vi "Set Double Complex.vi"(8 "error in":errorcluster, 9 "value":cdb, 10 "variable name":string, 11 "GOLPI ref. in":T1={"pipe handle"={"lv_proc.dll file path"=path "", "process instance handle"=[], "debug mode"=FALSE, "debug data"=[]}, "fast read timeout [ms]"=500, "fast read settle time [ms]"=10, "fast read to multiple [ms]"=1, "max elements per input line"=100, "slow read timeout [ms]"=5000, "stdin double format specifier"="%_16e", "max elements per stdout output column"=100, "console mode bitstream"=FALSE, "bitstream first read timeout [ms]"=1000, "bitstream read timeout [ms]"=50, "struct transfer possible"=FALSE, "matlab mode"=FALSE, "var pipe write timeout [ms]"=5000, "variable pipe mode"=FALSE, "variable pipe buffer size [Bytes]"=10000000, "variable pipe block size [Bytes]"=1000000} {"variable pipe block size [Bytes]" format="%.0p"; "variable pipe buffer size [Bytes]" format="%.0p"}) -> (0 "error out":errorcluster, 3 "GOLPI ref. out":T1={"pipe handle"={"lv_proc.dll file path"=path "", "process instance handle"=[], "debug mode"=FALSE, "debug data"=[]}, "fast read timeout [ms]"=500, "fast read settle time [ms]"=10, "fast read to multiple [ms]"=1, "max elements per input line"=100, "slow read timeout [ms]"=5000, "stdin double format specifier"="%_16e", "max elements per stdout output column"=100, "console mode bitstream"=FALSE, "bitstream first read timeout [ms]"=1000, "bitstream read timeout [ms]"=50, "struct transfer possible"=FALSE, "matlab mode"=FALSE, "var pipe write timeout [ms]"=5000, "variable pipe mode"=FALSE, "variable pipe buffer size [Bytes]"=10000000, "variable pipe block size [Bytes]"=1000000} {"variable pipe block size [Bytes]" format="%.0p"; "variable pipe buffer size [Bytes]" format="%.0p"})   [LabVIEW 2020, in "GOLPI library.lvlib"]
doc: "Part of polymorph Set Variable.vi"
uses:
  GOLPI library.lvlib
  Public/GOLPI reference Type Def.ctl
  LV Process source distribution/Pipe Handle.ctl
  LV Process source distribution/LV Process library.lvlib
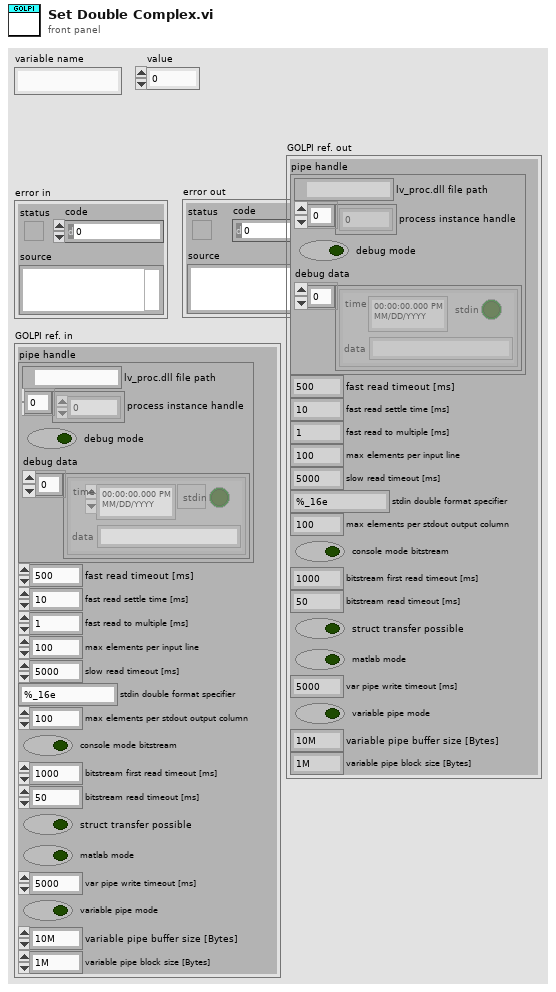
[diagram p1: front panel]
types:
  T1 = typedef "GOLPI library.lvlib/GOLPI reference Type Def.ctl" = cluster{"pipe handle":T2, "fast read timeout [ms]":u32, "fast read settle time [ms]":u32, "fast read to multiple [ms]":u32, "max elements per input line":u32, "slow read timeout [ms]":u32, "stdin double format specifier":string, "max elements per stdout output column":u32, "console mode bitstream":bool, "bitstream first read timeout [ms]":u32, "bitstream read timeout [ms]":u32, "struct transfer possible":bool, "matlab mode":bool, "var pipe write timeout [ms]":u32, "variable pipe mode":bool, "variable pipe buffer size [Bytes]":u32, "variable pipe block size [Bytes]":u32}
  T2 = typedef "LV Process library.lvlib/Pipe Handle.ctl" = cluster{"lv_proc.dll file path":path, "process instance handle":u32[], "debug mode":bool, "debug data":cluster{"time":timestamp, "stdin":bool, "data":string}[]}
  T3 = typedef "GOLPI library.lvlib/Transfer Mode.ctl" = enum16{"Matlab", "stdio", "temp file", "bitstream", "pipe"}
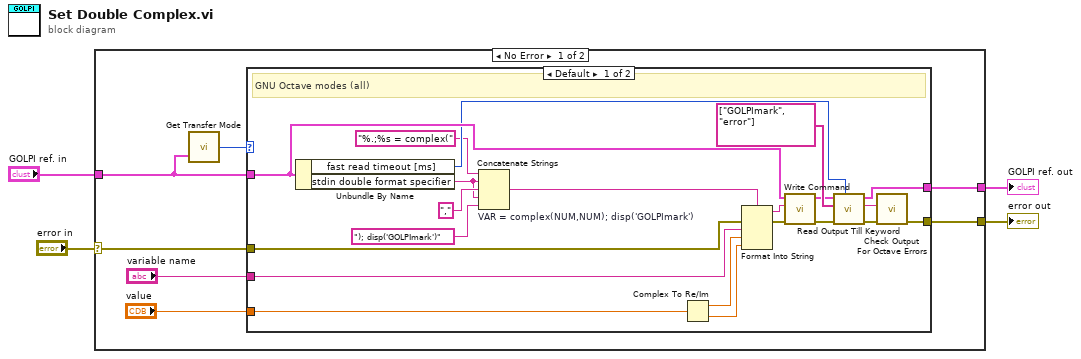
[diagram p0: block diagram]
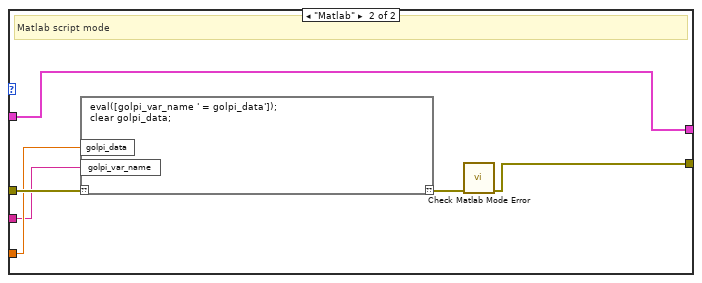
[diagram p2: hidden frame]
diagram:
  n1 = case shown="No Error" "error in" {
    selector: "error in" -> [w11 w40]
    tunnel: [w10 w40] -> w4
    tunnel: "GOLPI ref. in" -> [w6 w39]
    tunnel: [w9 w39] -> w1
    frame No Error {
      n2 = call "Get Transfer Mode.vi"("GOLPI ref."=w6) -> ("mode"=w5:T3)  [unwired: 1 in]
      n3 = case shown="Default" w5 {
        tunnel: w11 -> [w32 w38]
        tunnel: [w24 w33] -> w10
        tunnel: [w21 w37] -> w9
        tunnel: w6 -> [w20 w37]
        tunnel: "value" -> [w13 w36]
        tunnel: "variable name" -> [w12 w35]
        frame Default {
          # "GNU Octave modes (all)"
          n4 = Unbundle By Name(w20) -> ("fast read timeout [ms]"=w19:u32, "stdin double format specifier"=w15:string)
          n5 = Concatenate Strings "VAR = complex(NUM,NUM); disp('GOLPImark')"("%.;%s = complex(" ("format string"), w15, "," ("string"), w15, "); disp('GOLPImark')" ("format string")) -> (w14:string)
          n6 = Complex To Re/Im(x + iy=w13) -> (x=w23:dbl, y=w22:dbl)
          n7 = Format Into String(format string=w14, error in=w32, w12, w23, w22) -> (resulting string=w30:string, error out=w31:errorcluster)  [unwired: 1 in]
          n8 = call "Write Command.vi"("error in"=w31, "command"=w30, "GOLPI ref. in"=w20) -> ("error out"=w29:errorcluster, "GOLPI ref. out"=w26:T1)  [unwired: 7 in]
          n9 = call "Read Output Till Keyword.vi"("timeout [ms]"=w19, "error in"=w29, "keywords"=string[] ["GOLPImark", "error"], "GOLPI ref. in"=w26) -> ("error out"=w28:errorcluster, "read buffer"=w25:string, "GOLPI ref. out"=w21:T1)  [unwired: 4 in, 1 out]
          n10 = call "Check Output For Octave Errors.vi"("error in"=w28, "read buffer"=w25) -> ("error out"=w24:errorcluster)  [unwired: 9 in]
        }
        frame "Matlab" {
          # "Matlab script mode"
          n11 = script code="eval([golpi_var_name ' = golpi_data']);\nclear golpi_data;"("??"=w38, "golpi_var_name"=w35, "golpi_data"=w36) -> ("??"=w34:errorcluster)
          n12 = call "Check Matlab Mode Error.vi"("error in"=w34) -> ("error out"=w33:errorcluster)  [unwired: 10 in]
        }
      }
    }
    frame Error {
    }
  }
  "error out" <- w4
  "GOLPI ref. out" <- w1
